vi "SplitStringMultiple.vi"(0 "String":string, 7 "Substring lengths":i32[](array[numeric])) -> (4 "Substrings":string[](array[string]), 8 "Rest of string":string)   [LabVIEW 2017, in "GPString.lvlib"]
doc: "Splits <B>String</B> into <B>Substrings</B> of <B>Substring lengths</B> and returns the <B>Rest of string</B> if anything is left.\n\nThe <B>Substrings</B> are always taken from the start of <B>String</B>, and a negative value in the <B>Substring lengths</B> array denotes a number of characters to skip instead a length to extract. The latter makes it possible to skip certain parts of the <B>String</B> while traveling down it to extract the <B>Substrings</B> you want.\n\nExamples:\n\"20130807-fish\" [4,2,2] -> [\"2013\",\"08\",\"07\"] and \"-fish\" as rest string.\n\"2013-08-07-fish\" [4,-1,2,-1,2] -> [\"2013\",\"08\",\"07\"] and \"-fish\" as rest string.\n\nThis VI is inlined.\n\nSteen Schmidt\nGPower\n8/7 2013"
uses:
  GPString.lvlib
panel:
  # "Copyright © 2016\nGPower\nSee enclosed license file for terms and conditions"
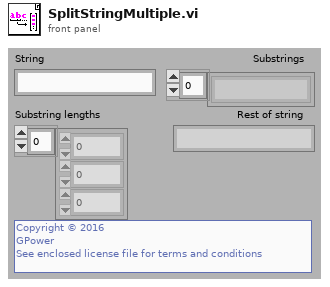
[diagram p1: front panel]
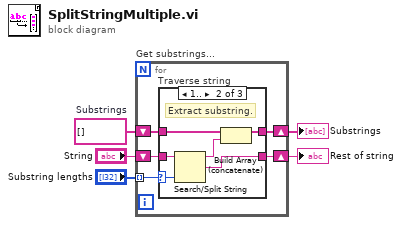
[diagram p0: block diagram]
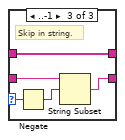
[diagram p3: hidden frame]
diagram:
  w2 = string[] []  # Substrings
  n1 = for "Get substrings..." {
    tunnel: "Substring lengths" -> [w8] mode=indexing
    shift-right: [w9] -> w3
    shift-left: "String" -> [w10]
    shift-right: [w6] -> w1
    shift-left: w2 -> [w7]
    n2 = case "Traverse string" shown="1.." w8 {
      selector: w8 -> [_ w16 w23]
      tunnel: w10 -> [w11 w18 w21]
      tunnel: [w11 w17 w19] -> w9
      tunnel: w7 -> [w12 w15 w22]
      tunnel: [w12 w13 w22] -> w6
      frame 0 {
      }
      frame 1.. {
        # "Extract substring."
        n3 = Search/Split String(string=w18, offset (0)=w16) -> (substring before match=w14:string, match + rest of string=w17:string)  [unwired: 1 in, 1 out]
        n4 = Build Array (concatenate)(w15, w14) -> (w13:string[])
      }
      frame ..-1 {
        # "Skip in string."
        n5 = Negate(x=w23) -> (-x=w20:i32)
        n6 = String Subset(string=w21, offset (0)=w20) -> (substring=w19:string)  [unwired: 1 in]
      }
    }
  }
  "Rest of string" <- w3
  "Substrings" <- w1
